vi "New Comm Interface.vi"(7 "Comm Interface in":refnum<class "Comm Interface.lvclass">, 8 "error in (no error)":errorcluster, 10 "Msg Update":refnum<user-event>, 11 "Connection Lst Enq":refnum<class "Message Enqueuer.lvclass">) -> (0 "error out":errorcluster, 3 "Comm Interface out":refnum<class "Comm Interface.lvclass">)   [LabVIEW 2017, in "Comm Interface.lvlib" / "Comm Interface.lvclass"]
uses:
  Comm Interface.lvclass
  <vilib>/ActorFramework/Message Enqueuer/Message Enqueuer.lvclass
  Comm Interface.lvclass/Comm Interface.ctl
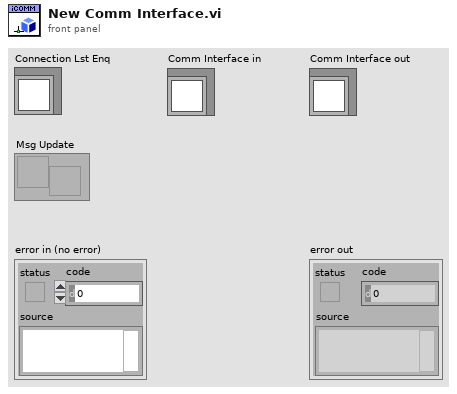
[diagram p1: front panel]
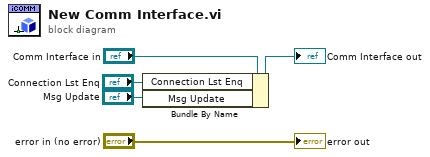
[diagram p0: block diagram]
diagram:
  n1 = Bundle By Name(cluster="Comm Interface in", "Connection Lst Enq"="Connection Lst Enq", "Msg Update"="Msg Update") -> (→"Comm Interface out":refnum<class "Comm Interface.lvclass">)
  "error out" <- "error in (no error)"
